vi "ToGraphML.vi"(8 "error in (no error)":errorcluster, 10 "file":path=path "C:/Users/bkinding/Desktop/soduku.xml", 11 "Graph in":refnum<class "Graph.lvclass">) -> (0 "error out":errorcluster, 3 "Graph out":refnum<class "Graph.lvclass">)   [LabVIEW 2010, in "Graph.lvclass"]
uses:
  Graph/Graph.lvclass
  Common/BasicSortedList/BasicSortedList/BasicSortedList.lvclass
  GraphNode/GraphNode.lvclass
  Graph/Read ClosedList.vi
  Graph/Read OpenList.vi
  LinkedList/LinkedList.lvclass
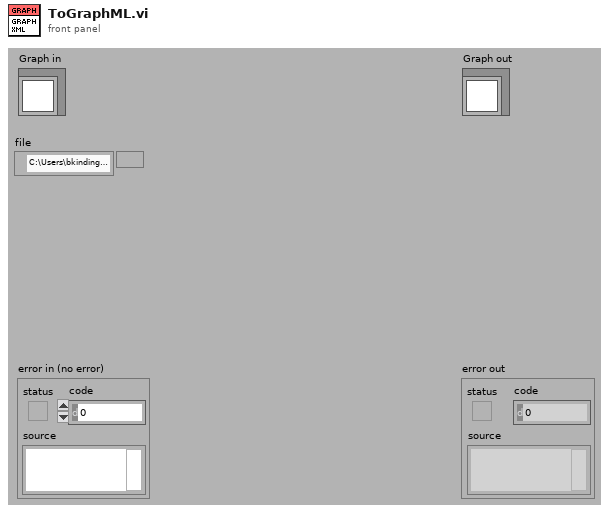
[diagram p1: front panel]
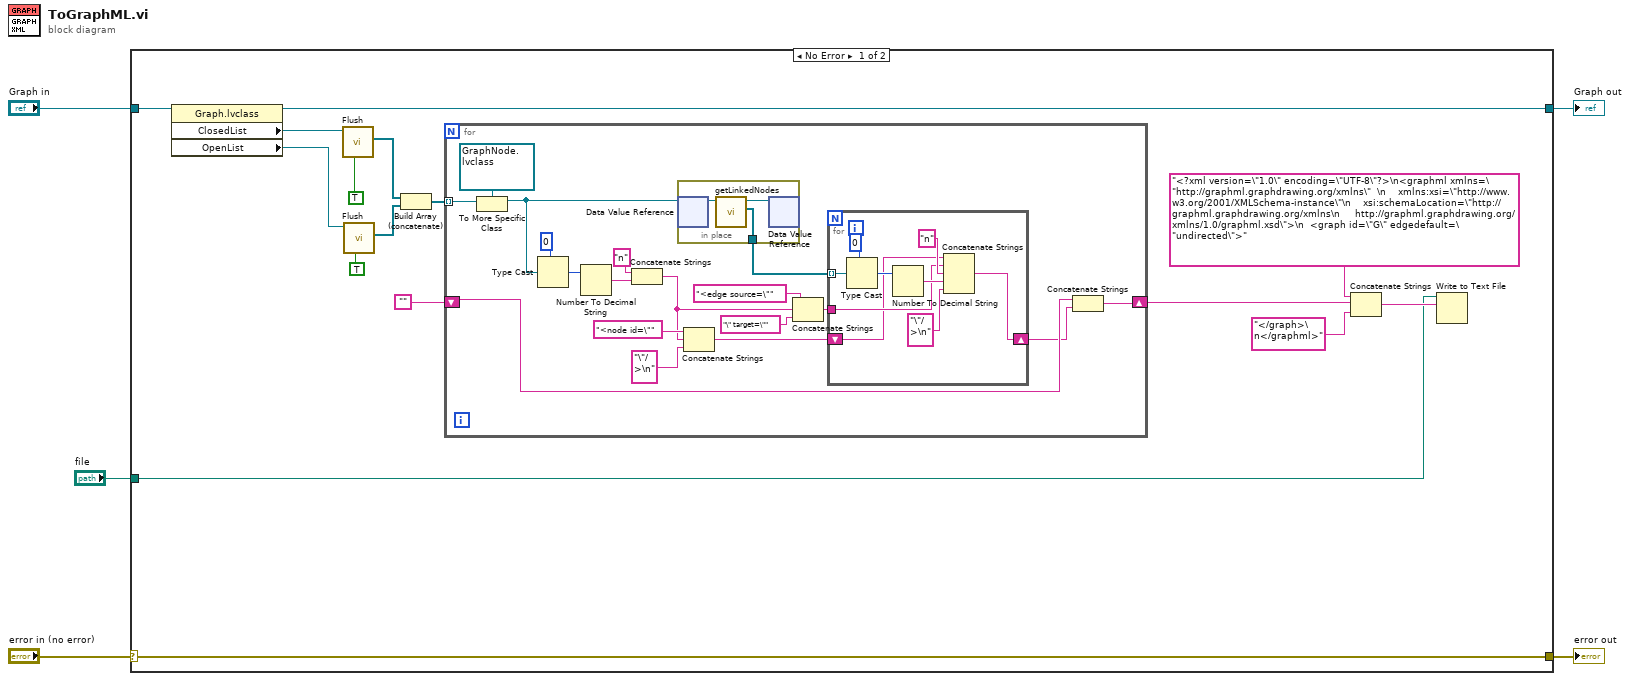
[diagram p0: block diagram]
diagram:
  n1 = case shown="No Error" "error in (no error)" {
    selector: "error in (no error)" -> [w21 w53]
    tunnel: [w21 w53] -> w4
    tunnel: [w19 w52] -> w2
    tunnel: "Graph in" -> [w20 w52]
    tunnel: "file" -> [w6 _]
    frame No Error {
      n2 = property class="Graph.lvclass"(reference=w20) -> (reference out=w19:refnum<class "Graph.lvclass">, "ClosedList"=w18:refnum<class "BasicSortedList.lvclass">, "OpenList"=w15:refnum<class "BasicSortedList.lvclass">)  [unwired: 1 in, 1 out]
      n3 = call "Flush.vi"("returnNodes"=TRUE, "LinkedList in"=w18) -> ("Nodes"=w14:refnum<data-value>[])  [unwired: 7 in, 2 out]
      n4 = call "Flush.vi"("returnNodes"=TRUE, "LinkedList in"=w15) -> ("Nodes"=w13:refnum<data-value>[])  [unwired: 7 in, 2 out]
      n5 = Build Array (concatenate)(w14, w13) -> (w12:refnum<data-value>[])
      n6 = for {
        tunnel: w12 -> [w39] mode=indexing
        shift-right: [w22] -> w9
        shift-left: "" -> [w24]
        n7 = To More Specific Class(target class=refnum<data-value> refnum ("data value reference"), reference=w39) -> (specific class reference=w37:refnum<data-value>)  [unwired: 1 in, 1 out]
        n8 = Type Cast(type=u32 0, x=w37) -> (*(type *) &x=w35:u32)
        n9 = Number To Decimal String(number=w35) -> (decimal integer string=w34:string)  [unwired: 1 in]
        n10 = Concatenate Strings("n", w34) -> (w27:string)
        n11 = in-place {
          in-place-border: [w49] -> w29
          n12 = in-place-dvr #1(w37) -> (w51:refnum<class "GraphNode.lvclass">)  [unwired: 1 out]
          n13 = call "getLinkedNodes.vi"("GraphNode in"=w51) -> ("LinkedNodes"=w49:refnum<data-value>[], "GraphNode out"=w50:refnum<class "GraphNode.lvclass">)  [unwired: 8 in, 1 out]
          n14 = in-place-dvr #1(w50) -> ()  [unwired: 2 out]
        }
        n15 = Concatenate Strings("<node id=\"", w27, "\"/>\n") -> (w30:string)
        n16 = Concatenate Strings("<edge source=\"", w27, "\" target=\"") -> (w25:string)
        n17 = for {
          shift-right: [w40] -> w23
          shift-left: w30 -> [w41]
          tunnel: w29 -> [w44] mode=indexing
          tunnel: w25 -> [w43]
          n18 = Type Cast(type=u32 0, x=w44) -> (*(type *) &x=w47:u32)
          n19 = Number To Decimal String(number=w47) -> (decimal integer string=w46:string)  [unwired: 1 in]
          n20 = Concatenate Strings(w41, w43, "n", w46, "\"/>\n") -> (w40:string)
        }
        n21 = Concatenate Strings(w24, w23) -> (w22:string)
      }
      n22 = Concatenate Strings("<?xml version=\"1.0\" encoding=\"UTF-8\"?>\n<graphml xmlns=\"http://graphml.graphdrawing.org/xmlns\"  \n    xmlns:xsi=\"http://www.w3.org/2001/XMLSchema-instance\"\n    xsi:schemaLocation=\"http://graphml.graphdrawing.org/xmlns\n     http://graphml.graphdrawing.org/xmlns/1.0/graphml.xsd\">\n  <graph id=\"G\" edgedefault=\"undirected\">", w9, "</graph>\n</graphml>") -> (w7:string)
      n23 = Write to Text File(file (use dialog)=w6, text=w7) -> ()  [unwired: 2 in, 3 out]
    }
    frame Error {
    }
  }
  "error out" <- w4
  "Graph out" <- w2
